vi "2D String To 1D I32.vi"(10 "2D String In":string[][](array[string])) -> (2 "1D I32":i32[](array[numeric]))   [LabVIEW 2024]
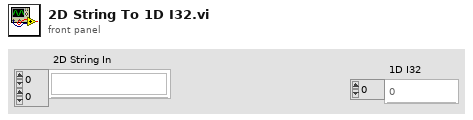
[diagram p1: front panel]
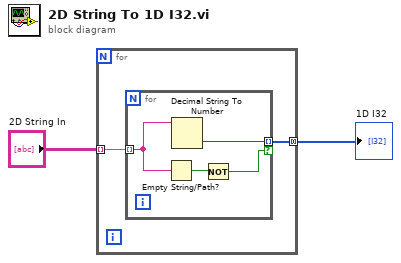
[diagram p0: block diagram]
diagram:
  n1 = for {
    tunnel: "2D String In" -> [w4] mode=indexing
    tunnel: [w3] -> w1 mode=concatenating
    n2 = for {
      tunnel: w4 -> [w8] mode=indexing
      tunnel: [w6] -> w3 mode=indexing if=w5
      n3 = Empty String/Path?(string/path=w8) -> (empty?=w7:bool)
      n4 = Decimal String To Number(string=w8) -> (number=w6:i32)  [unwired: 2 in, 1 out]
      n5 = Not(x=w7) -> (.not. x?=w5:bool)
    }
  }
  "1D I32" <- w1
